vi "Master Setup Export.vi"(5 "Export all files?":bool, 7 "Zip File Path":path, 9 "Master Setup Path":path, 10 "Setup Files":string[](array[string]), 11 "Setup File Paths":path[](array[path])) -> ()   [LabVIEW 2017]
panel:
  in  "Cancel":bool
  in  "OK":bool
  in  "Add":bool
  in  "Remove":bool
  in  "Files to Export":i32(listbox)
  in  "Files Available":i32[](listbox)
  # "REPS Export Setup Utility"
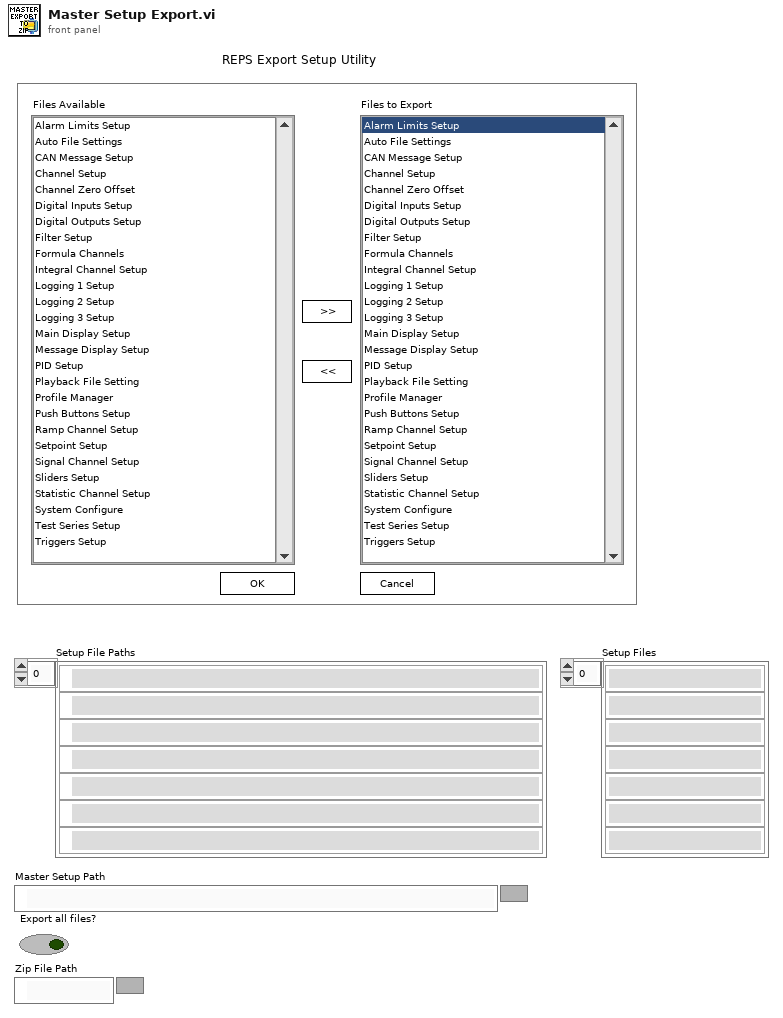
[diagram p1: front panel]
types:
  T1 = enum16{"open", "replace", "create", "open or create", "replace or create", "replace or create with confirmation"}
  T2 = cluster{"Export File Paths":path[], "Files":string, "Zip File Path":path}
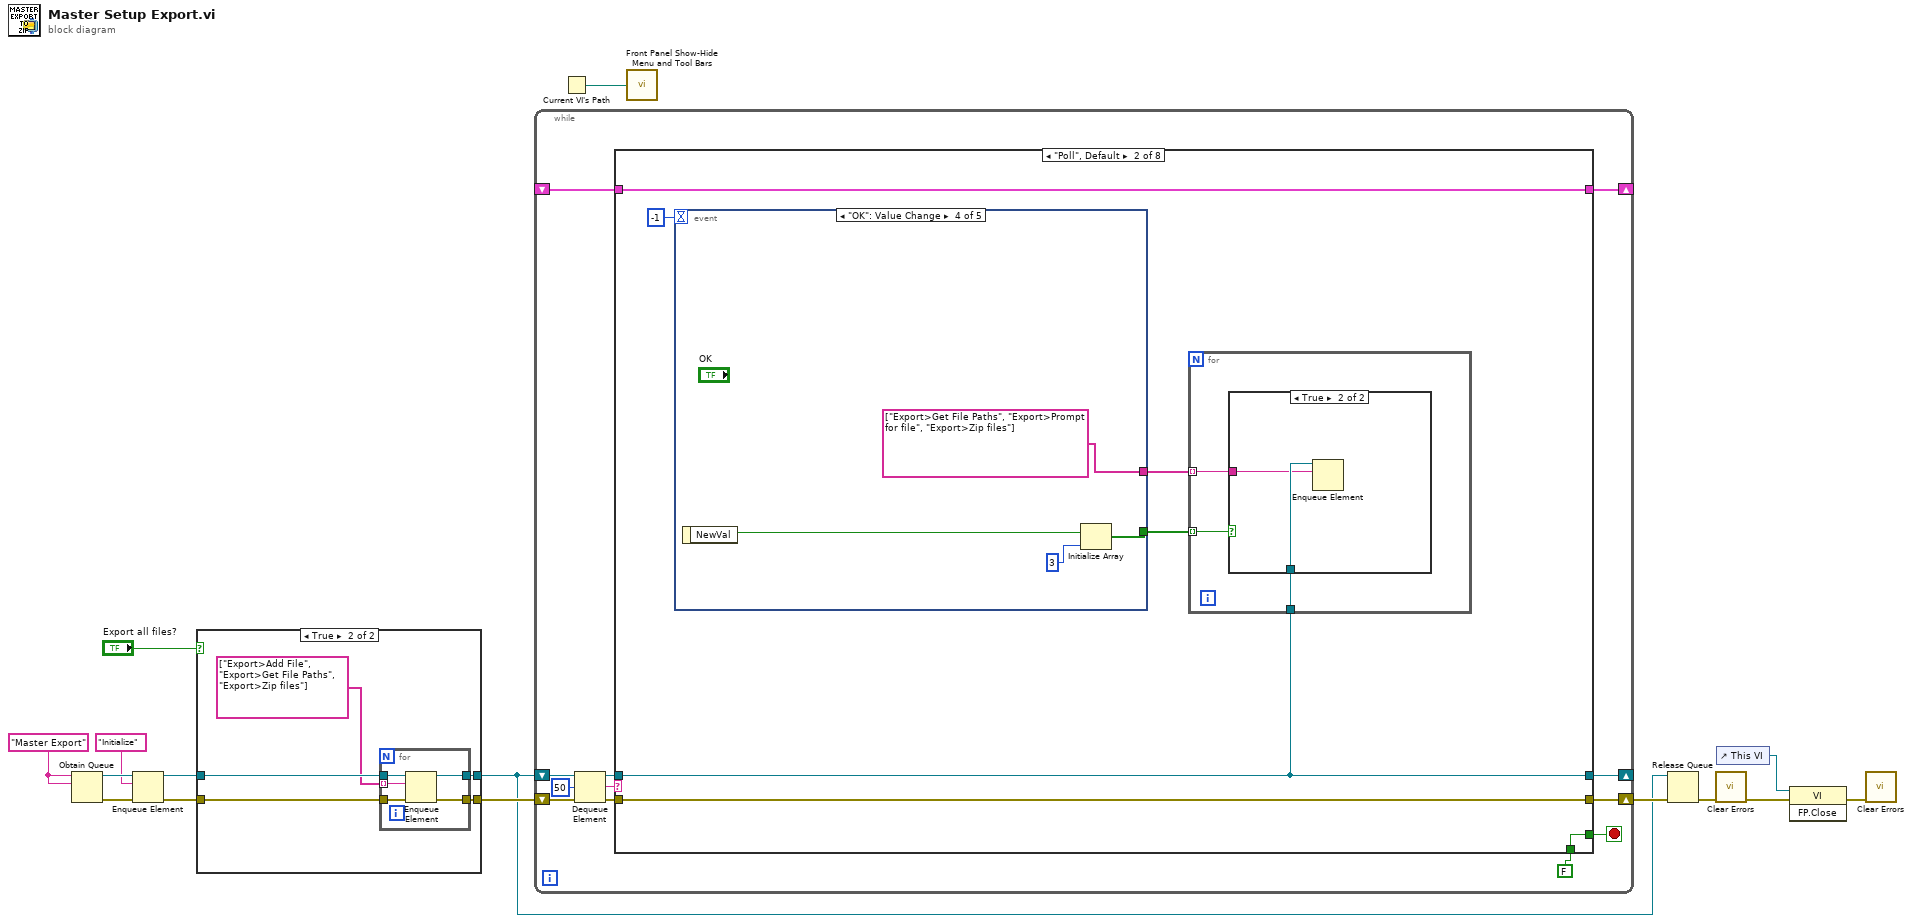
[diagram p0: block diagram]
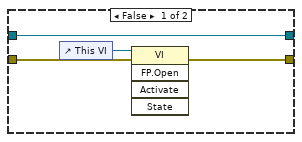
[diagram p2: hidden frame]
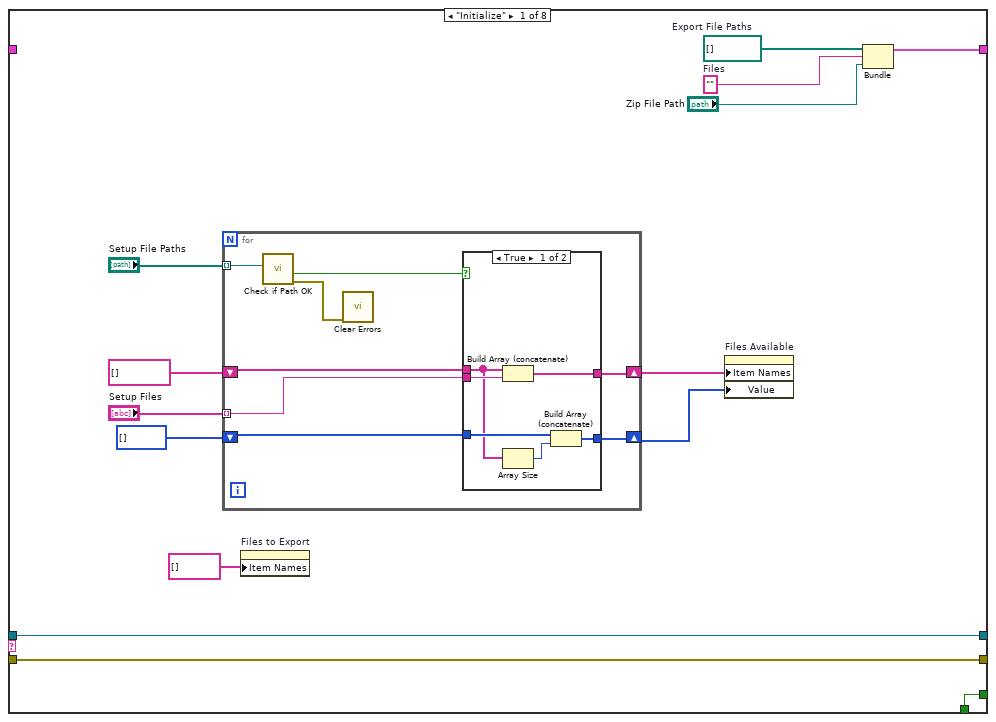
[diagram p3: hidden frame]
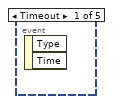
[diagram p6: hidden frame]
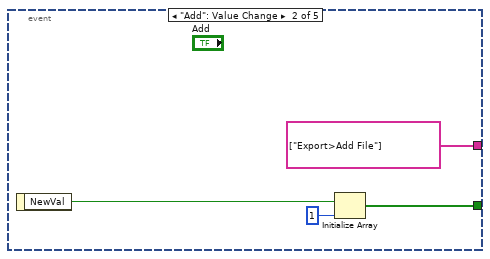
[diagram p7: hidden frame]
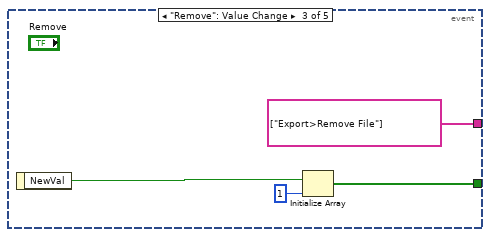
[diagram p8: hidden frame]
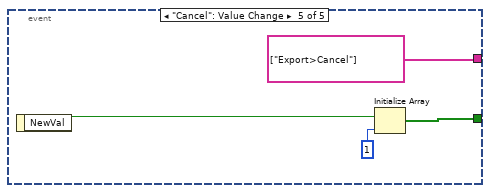
[diagram p9: hidden frame]
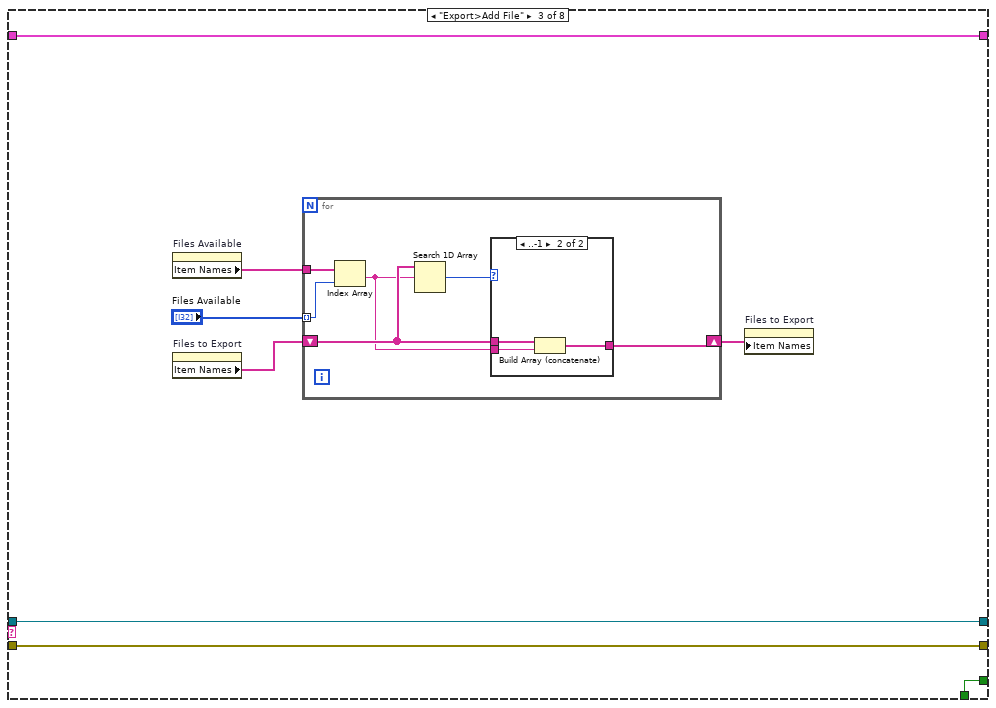
[diagram p10: hidden frame]
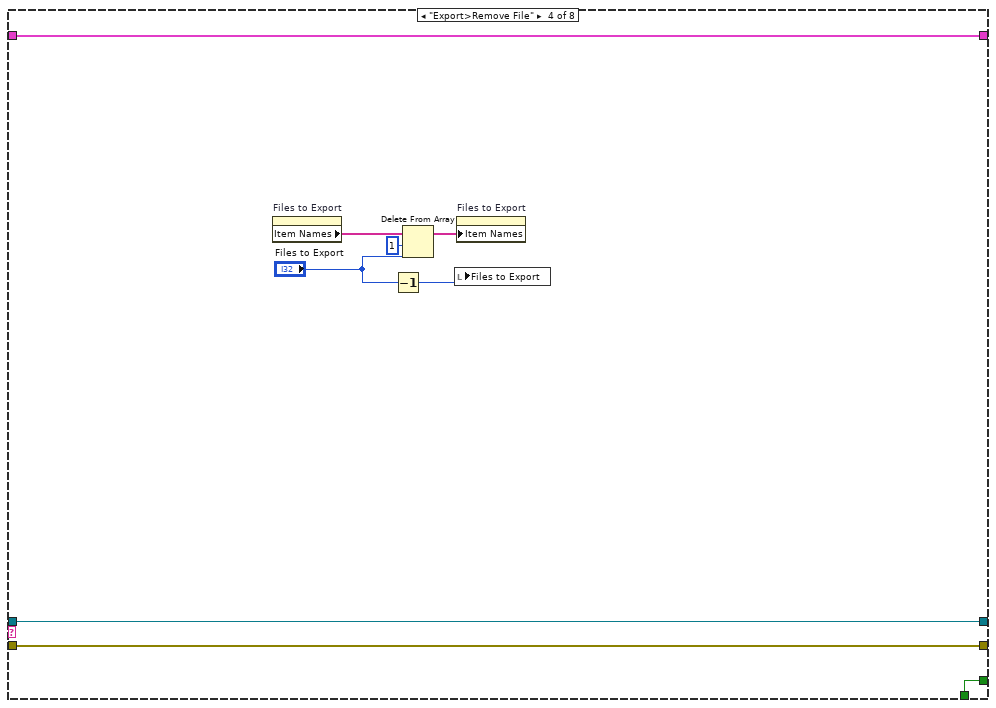
[diagram p12: hidden frame]
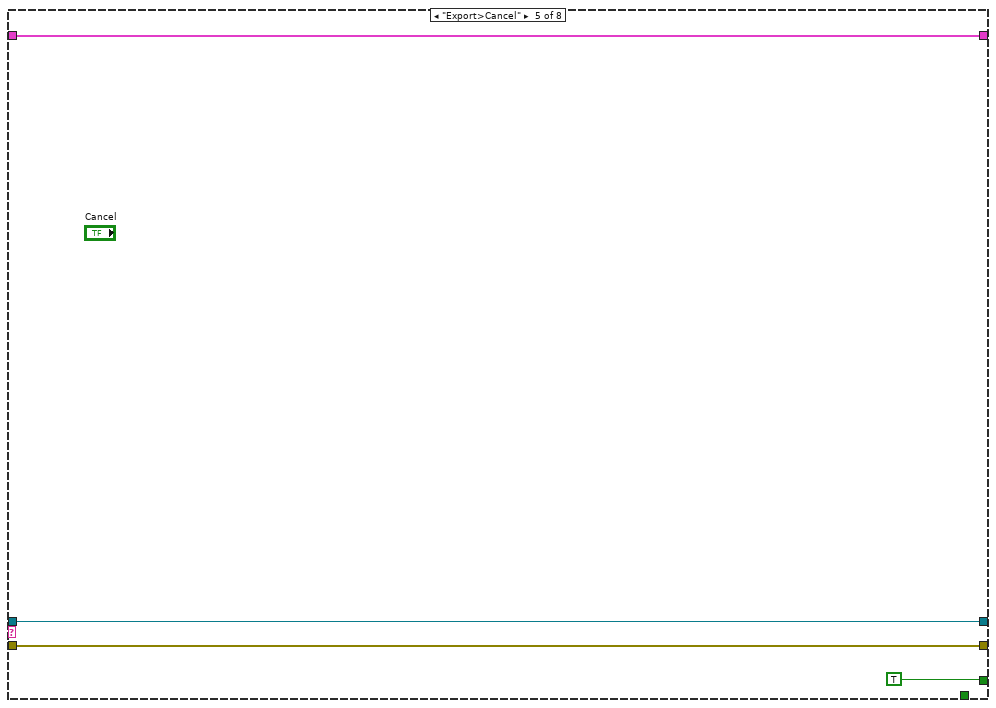
[diagram p13: hidden frame]
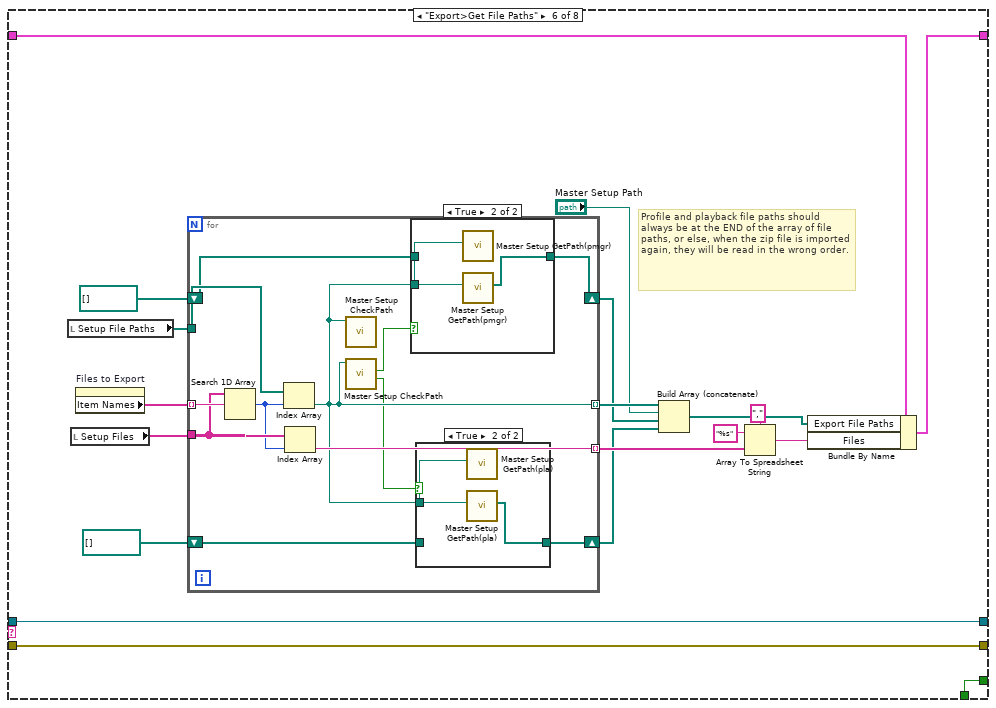
[diagram p14: hidden frame]
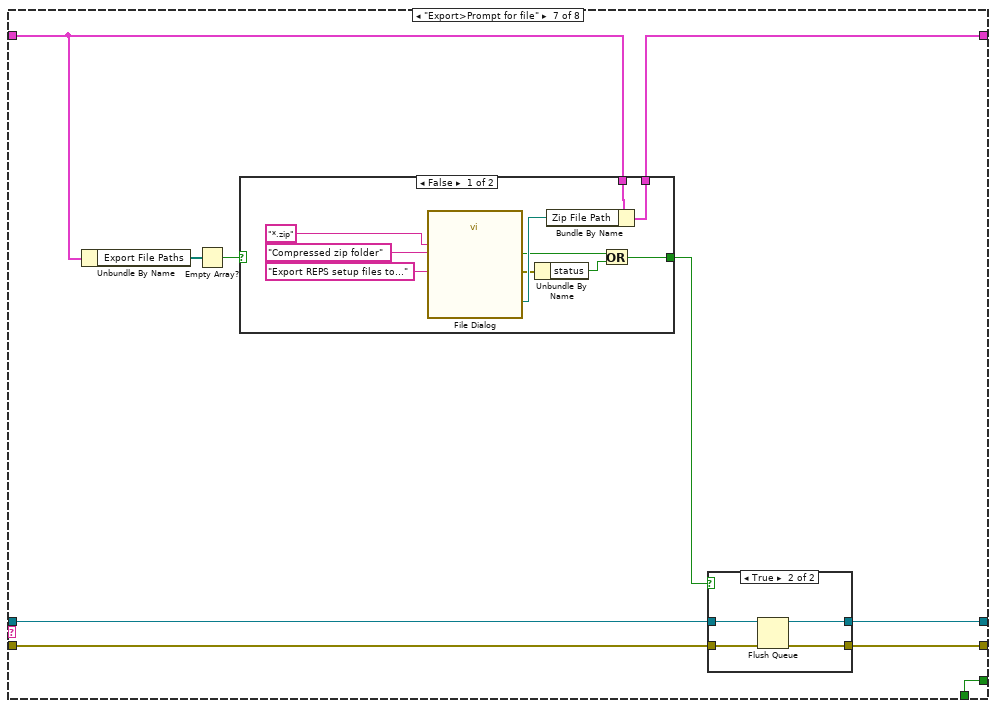
[diagram p17: hidden frame]
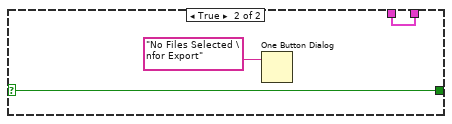
[diagram p18: hidden frame]
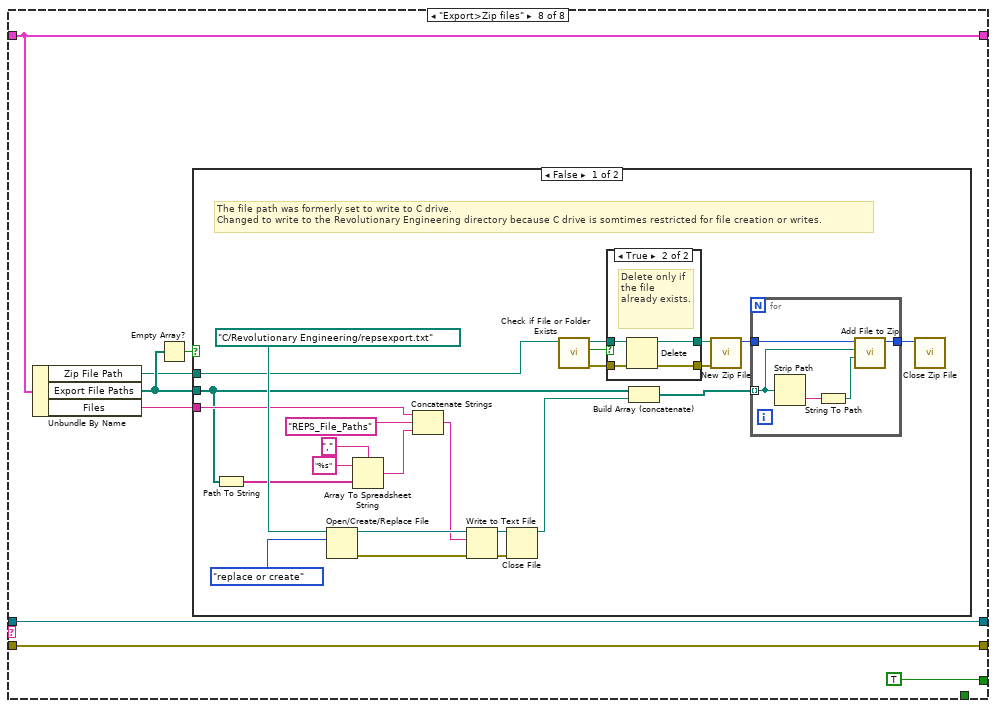
[diagram p20: hidden frame]
diagram:
  w15 = "Master Export" ("name (unnamed)")
  n1 = Obtain Queue(name (unnamed)=w15, element data type=w15) -> (queue out=w14:refnum<queue>, error out=w12:errorcluster)  [unwired: 3 in, 1 out]
  n2 = Enqueue Element(queue=w14, element="Initialize" ("name (unnamed)"), error in (no error)=w12) -> (queue out=w5:refnum<queue>, error out=w4:errorcluster)  [unwired: 1 in, 1 out]
  n3 = case shown="True" "Export all files?" {
    tunnel: w5 -> [w19 w24]
    tunnel: w4 -> [w17 w23]
    tunnel: [w16 w22] -> w3
    tunnel: [w19 w21] -> w2
    frame False {
      n4 = control-ref of="This VI"() -> (w18:refnum<vi>)
      n5 = invoke class="VI" method="FP.Open"(reference=w18, error in=w17) -> (error out=w16:errorcluster)  [unwired: 3 in, 4 out]
    }
    frame True {
      n6 = for {
        tunnel: w24 -> [w29]
        tunnel: w23 -> [w28]
        tunnel: [w27] -> w22
        tunnel: [w26] -> w21
        tunnel: string[] ["Export>Add File", "Export>Get File Paths", "Export>Zip files"] -> [w25] mode=indexing
        n7 = Enqueue Element(queue=w29, element=w25, error in (no error)=w28) -> (queue out=w26:refnum<queue>, error out=w27:errorcluster)  [unwired: 1 in, 1 out]
      }
    }
  }
  n8 = while {
    shift-right: [w36] -> _
    shift-left: w2 -> [w41]
    shift-right: [w35] -> w10
    shift-left: w3 -> [w38]
    shift-right: [w31] -> _
    shift-left: _ -> [w30]
    stop <- w33 stop-if-true
    n9 = Dequeue Element(queue=w41, timeout in ms (-1)=50, error in (no error)=w38) -> (queue out=w40:refnum<queue>, element=w39:string, error out=w37:errorcluster)  [unwired: 1 out]
    n10 = case shown="\"Poll\", Default" w39 {
      tunnel: w40 -> [w43 w73 w107 w126 w130 w146 w175 w202]
      tunnel: w37 -> [w42 w78 w106 w125 w129 w145 w174 w203]
      tunnel: [w43 w73 w107 w126 w130 w146 w173 w202] -> w36
      tunnel: [w42 w78 w106 w125 w129 w145 w172 w203] -> w35
      tunnel: [w55 w77 w105 w124 TRUE w144 w177 TRUE] -> w33
      tunnel: FALSE -> [w55 w77 w105 w124 _ w144 w177 _]
      tunnel: [w50 w72 w102 w120 w127 w142 w176 w204] -> w31
      tunnel: w30 -> [_ w72 w102 w120 w127 w143 w170 w204]
      frame "Initialize" {
        w49 = path[] []  # Export File Paths
        w45 = ""  # Files
        n11 = for {
          tunnel: "Setup File Paths" -> [w58] mode=indexing
          shift-right: [w62] -> w48
          shift-left: string[] [] -> [w63]
          tunnel: "Setup Files" -> [w61] mode=indexing
          shift-right: [w59] -> w46
          shift-left: i32[] [] -> [w60]
          n12 = call "Check if Path OK.vi"("Path"=w58) -> ("error out"=w56:errorcluster, "Path OK"=w57:bool)  [unwired: 8 in, 1 out]
          n13 = call <vilib>:"Clear Errors.vi"("error in (no error)"=w56) -> ()  [unwired: 5 in, 2 out]
          n14 = case shown="True" w57 {
            tunnel: w63 -> [w65 w71]
            tunnel: [w69 w71] -> w62
            tunnel: w61 -> [w68 _]
            tunnel: w60 -> [w67 w70]
            tunnel: [w66 w70] -> w59
            frame True {
              n15 = Build Array (concatenate)(w65, w68) -> (w69:string[])
              n16 = Array Size(array=w65) -> (size(s)=w64:i32)
              n17 = Build Array (concatenate)(w67, w64) -> (w66:i32[])
            }
            frame False {
            }
          }
        }
        n18 = property on="Files to Export" class="LstBox (strict)"("Item Names"=string[] []) -> ()  [unwired: 2 in, 2 out]
        n19 = property on="Files Available" class="LstBox (strict)"("Item Names"=w48, "Value"=w46) -> ()  [unwired: 2 in, 2 out]
        n20 = Bundle("Export File Paths"=w49, "Files"=w45, "Zip File Path"="Zip File Path") -> (w50:T2)  [unwired: 1 in]
      }
      frame "Poll", Default {
        n21 = event shown="[3] \"OK\": Value Change" {
          selector: _ -> [_ _ _ _ _]
          dyn-events: _ -> [_ _ _ _ _]
          timeout: -1 -> [_ _ _ _ _]
          tunnel: [_ string[] ["Export>Add File"] string[] ["Export>Remove File"] string[] ["Export>Get File Paths", "Export>Prompt for file", "Export>Zip files"] string[] ["Export>Cancel"]] -> w75
          tunnel: [_ w85 w89 w93 w98] -> w74
          event Timeout {
            n22 = event-data() -> ()  [unwired: 1 in, 2 out]
          }
          event "Add": Value Change {
            n23 = event-data() -> ("NewVal"=w86:bool)  [unwired: 1 in]
            n24 = Initialize Array(w86, 1 ("dimension size")) -> (w85:bool[])
          }
          event "Remove": Value Change {
            n25 = event-data() -> ("NewVal"=w88:bool)  [unwired: 1 in]
            n26 = Initialize Array(w88, 1 ("dimension size")) -> (w89:bool[])
          }
          event "OK": Value Change {
            n27 = event-data() -> ("NewVal"=w94:bool)  [unwired: 1 in]
            n28 = Initialize Array(w94, 3 ("dimension size")) -> (w93:bool[])
          }
          event "Cancel": Value Change {
            n29 = event-data() -> ("NewVal"=w97:bool)  [unwired: 1 in]
            n30 = Initialize Array(w97, 1 ("dimension size")) -> (w98:bool[])
          }
        }
        n31 = for {
          tunnel: w75 -> [w81] mode=indexing
          tunnel: w74 -> [w80] mode=indexing
          tunnel: w73 -> [w79]
          n32 = case shown="True" w80 {
            tunnel: w81 -> [_ w82]
            tunnel: w79 -> [_ w83]
            frame False {
            }
            frame True {
              n33 = Enqueue Element(queue=w83, element=w82) -> ()  [unwired: 2 in, 3 out]
            }
          }
        }
      }
      frame "Export>Add File" {
        n34 = property on="Files Available" class="LstBox (strict)"() -> ("Item Names"=w103:string[])  [unwired: 2 in, 2 out]
        n35 = property on="Files to Export" class="LstBox (strict)"() -> ("Item Names"=w101:string[])  [unwired: 2 in, 2 out]
        n36 = for {
          tunnel: "Files Available" -> [w112] mode=indexing
          tunnel: w103 -> [w113]
          shift-right: [w108] -> w100
          shift-left: w101 -> [w110]
          n37 = Index Array(array=w113, index=w112) -> (element=w109:string)
          n38 = Search 1D Array(1D array=w110, element=w109) -> (index of element=w111:i32)  [unwired: 1 in]
          n39 = case shown="..-1" w111 {
            tunnel: w110 -> [w114 w117]
            tunnel: w109 -> [_ w116]
            tunnel: [w114 w115] -> w108
            frame 0.. {
            }
            frame ..-1 {
              n40 = Build Array (concatenate)(w117, w116) -> (w115:string[])
            }
          }
        }
        n41 = property on="Files to Export" class="LstBox (strict)"("Item Names"=w100) -> ()  [unwired: 2 in, 2 out]
      }
      frame "Export>Remove File" {
        n42 = property on="Files to Export" class="LstBox (strict)"() -> ("Item Names"=w123:string[])  [unwired: 2 in, 2 out]
        n43 = Decrement(x="Files to Export") -> (x-1=w118:i32)
        n44 = Delete From Array(array=w123, length=1, index="Files to Export") -> (array with subset deleted=w121:string[])  [unwired: 1 out]
        n45 = local write "Files to Export"(w118) -> ()
        n46 = property on="Files to Export" class="LstBox (strict)"("Item Names"=w121) -> ()  [unwired: 2 in, 2 out]
      }
      frame "Export>Cancel" {
      }
      frame "Export>Get File Paths" {
        # "Profile and playback file paths should always be at the END of the array of file paths, or else, when the zip file is imported again, they will be read in the wrong order."
        n47 = local read "Setup File Paths"() -> (w147:path[])
        n48 = local read "Setup Files"() -> (w148:string[])
        n49 = property on="Files to Export" class="LstBox (strict)"() -> ("Item Names"=w149:string[])  [unwired: 2 in, 2 out]
        n50 = for {
          tunnel: w149 -> [w161] mode=indexing
          tunnel: w148 -> [w159]
          tunnel: w147 -> [w160]
          tunnel: [w157] -> w141 mode=indexing
          tunnel: [w156] -> w135 mode=indexing
          shift-right: [w155] -> w134
          shift-left: path[] [] ("path array") -> [w154]
          shift-right: [w153] -> w133
          shift-left: path[] [] ("path array") -> [w152]
          n51 = Search 1D Array(1D array=w159, element=w161) -> (index of element=w158:i32)  [unwired: 1 in]
          n52 = Index Array(array=w160, index=w158) -> (element=w156:path)
          n53 = Index Array(array=w159, index=w158) -> (element=w157:string)
          n54 = call "Master Setup CheckPath.vi"("filepath"=w156) -> ()  [unwired: 7 in, 4 out]
          n55 = call "Master Setup CheckPath.vi"("filepath"=w156) -> ("pla available?"=w151:bool, "pmgr available?"=w150:bool)  [unwired: 7 in, 2 out]
          n56 = case shown="True" w150 {
            tunnel: w156 -> [_ w167]
            tunnel: [w165 w166] -> w155
            tunnel: w154 -> [w165 _]
            frame False {
            }
            frame True {
              n57 = call "Master Setup GetPath(pmgr).vi"("path in"=w167) -> ()  [unwired: 10 in, 1 out]
              n58 = call "Master Setup GetPath(pmgr).vi"("path in"=w167) -> ("path array"=w166:path[])  [unwired: 10 in]
            }
          }
          n59 = case shown="True" w151 {
            tunnel: w156 -> [_ w164]
            tunnel: [w162 w163] -> w153
            tunnel: w152 -> [w162 _]
            frame False {
            }
            frame True {
              n60 = call "Master Setup GetPath(pla).vi"("path in"=w164) -> ()  [unwired: 10 in, 1 out]
              n61 = call "Master Setup GetPath(pla).vi"("path in"=w164) -> ("path array"=w163:path[])  [unwired: 10 in]
            }
          }
        }
        n62 = Build Array (concatenate)(w135, "Master Setup Path", w134, w133) -> (w132:path[])
        n63 = Array To Spreadsheet String(delimiter (Tab)=",", array=w141, 3:"%s" ("format string")) -> (spreadsheet string=w140:string)
        n64 = Bundle By Name(cluster=w143, "Export File Paths"=w132, "Files"=w140) -> (w142:T2)
      }
      frame "Export>Prompt for file" {
        n65 = Unbundle By Name(w170) -> ("Export File Paths"=w169:path[])
        n66 = Empty Array?(array=w169) -> (empty?=w168:bool)
        n67 = case shown="False" w168 {
          selector: w168 -> [_ w188]
          tunnel: [w186 w190] -> w176
          tunnel: [w185 w188] -> w171
          tunnel: w170 -> [w184 w190]
          frame False {
            n68 = call "File Dialog"("prompt"="Export REPS setup files to...", "pattern (all files)"="*.zip", "pattern label"="Compressed zip folder") -> ("selected path"=w183:path, "cancelled"=w182:bool, "error out"=w181:errorcluster)  [unwired: 9 in, 1 out]
            n69 = Unbundle By Name(w181) -> ("status"=w187:bool)
            n70 = Bundle By Name(cluster=w184, "Zip File Path"=w183) -> (w186:T2)
            n71 = Or(x=w182, y=w187) -> (x .or. y?=w185:bool)
          }
          frame True {
            n72 = One Button Dialog(message="No Files Selected \nfor Export") -> ()  [unwired: 1 in, 1 out]
          }
        }
        n73 = case shown="True" w171 {
          tunnel: w175 -> [w192 w196]
          tunnel: w174 -> [w191 w195]
          tunnel: [w192 w194] -> w173
          tunnel: [w191 w193] -> w172
          frame False {
          }
          frame True {
            n74 = Flush Queue(queue=w196, error in (no error)=w195) -> (queue out=w194:refnum<queue>, error out=w193:errorcluster)  [unwired: 1 out]
          }
        }
      }
      frame "Export>Zip files" {
        n75 = Unbundle By Name(w204) -> ("Zip File Path"=w197:path, "Export File Paths"=w198:path[], "Files"=w199:string)
        n76 = Empty Array?(array=w198) -> (empty?=w200:bool)
        n77 = case shown="False" w200 {
          tunnel: w198 -> [w206 _]
          tunnel: w199 -> [w218 _]
          tunnel: w197 -> [w215 _]
          frame False {
            # "The file path was formerly set to write to C drive.\nChanged to write to the Revolutionary Engineering directory because C drive is somtimes restricted for file creation or writes."
            n78 = Path To String(path=w206) -> (string=w205:string[])
            n79 = Open/Create/Replace File(file path (use dialog)=path "C:/Revolutionary Engineering/repsexport.txt" ("file (use dialog)"), operation (0:open)=T1."replace or create") -> (refnum out=w224:refnum<file>, error out=w222:errorcluster)  [unwired: 4 in, 1 out]
            n80 = Array To Spreadsheet String(delimiter (Tab)=",", array=w205, 3:"%s" ("format string")) -> (spreadsheet string=w217:string)
            n81 = Concatenate Strings(w218, "REPS_File_Paths", w217) -> (w216:string)
            n82 = Write to Text File(file (use dialog)=w224, text=w216, error in=w222) -> (refnum out=w228:refnum<file>, error out=w226:errorcluster)  [unwired: 1 in, 1 out]
            n83 = Close File(refnum=w228, error in=w226) -> (path=w227:path)  [unwired: 1 out]
            n84 = call <vilib>:"Check if File or Folder Exists.vi"("path"=w215) -> ("error out"=w209:errorcluster, "file or folder exists?"=w211:bool, "dup path"=w210:path)  [unwired: 8 in]
            n85 = case shown="True" w211 {
              tunnel: w210 -> [w229 w234]
              tunnel: w209 -> [w230 w233]
              tunnel: [w230 w232] -> w208
              tunnel: [w229 w231] -> w207
              frame False {
              }
              frame True {
                # "Delete only if the file already exists."
                n86 = Delete(path (use dialog)=w234, error in=w233) -> (deleted path=w231:path, error out=w232:errorcluster)  [unwired: 3 in, 1 out]
              }
            }
            n87 = Build Array (concatenate)(w206, w227) -> (w212:path[])
            n88 = call <vilib>:"New Zip File.vi"("error in (no error)"=w208, "target"=w207) -> ("zip file out"=w214:i64)  [unwired: 3 in, 2 out]
            n89 = for {
              tunnel: w214 -> [w237]
              tunnel: w212 -> [w236] mode=indexing
              tunnel: [w235] -> w213
              n90 = Strip Path(path=w236) -> (name=w238:string)  [unwired: 1 out]
              n91 = String To Path(string=w238) -> (path=w239:path)
              n92 = call <vilib>:"Add File to Zip.vi"("destination path in zip"=w239, "source file path"=w236, "zip file in"=w237) -> ("zip file out"=w235:i64)  [unwired: 7 in, 1 out]
            }
            n93 = call <vilib>:"Close Zip File.vi"("zip file in"=w213) -> ()  [unwired: 6 in, 1 out]
          }
          frame True {
          }
        }
      }
    }
  }
  n94 = Current VI's Path() -> (path=w11:path)
  n95 = call "Front Panel Show-Hide Menu and Tool Bars.vi"("Current VI Path"=w11) -> ()  [unwired: 1 out]
  n96 = Release Queue(queue=w2, error in (no error)=w10) -> (error out=w9:errorcluster)  [unwired: 1 in, 2 out]
  n97 = call <vilib>:"Clear Errors.vi"("error in (no error)"=w9) -> ("error out"=w7:errorcluster)  [unwired: 5 in, 1 out]
  n98 = control-ref of="This VI"() -> (w8:refnum<vi>)
  n99 = invoke class="VI" method="FP.Close"(reference=w8, error in=w7) -> (error out=w1:errorcluster)  [unwired: 1 in, 2 out]
  n100 = call <vilib>:"Clear Errors.vi"("error in (no error)"=w1) -> ()  [unwired: 5 in, 2 out]
